vi "Read OTDComp.vi"(8 "error in (no error)":errorcluster, 11 "9212 in":refnum<class "9212.lvclass">) -> (0 "error out":errorcluster, 2 "OTDComp":bool, 3 "9212 out":refnum<class "9212.lvclass">)   [LabVIEW 2020, in "Modules.lvlib" / "9212.lvclass"]
uses:
  9212.lvclass
  9212.lvclass/9212.ctl
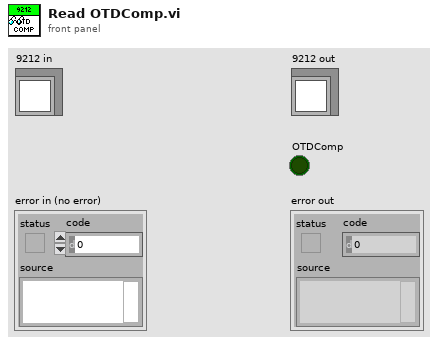
[diagram p1: front panel]
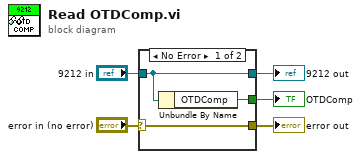
[diagram p0: block diagram]
diagram:
  n1 = case shown="No Error" "error in (no error)" {
    selector: "error in (no error)" -> [w8 w9]
    tunnel: [w8 w9] -> w4
    tunnel: [w7 w10] -> w2
    tunnel: "9212 in" -> [w7 w10]
    tunnel: [w6 _] -> w1
    frame No Error {
      n2 = Unbundle By Name(w7) -> ("OTDComp"=w6:bool)
    }
    frame Error {
    }
  }
  "error out" <- w4
  "9212 out" <- w2
  "OTDComp" <- w1
